vi "startTest.vi"(8 "error in (no error)":errorcluster, 10 "test":refnum<class>, 11 "TestResult in":refnum<class "TestResult.lvclass">) -> (0 "error out":errorcluster, 3 "TestResult in":refnum<class "TestResult.lvclass">)   [LabVIEW 2013, in "TestResult.lvclass"]
uses:
  TestResult.lvclass
  testStarted--Cluster.ctl
  TestResult.lvclass/TestResult.ctl
panel:
  # "JKI VI Tester for LabVIEW\nhttp://jkisoft.com/vi-tester\nCopyright (C) 2007-2009, JKI <info@jkisoft.com>\nALL RIGHTS RESERVED"
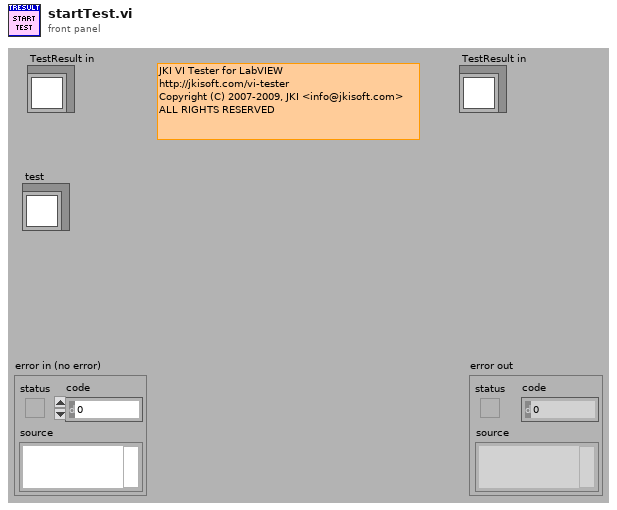
[diagram p1: front panel]
types:
  T1 = typedef "TestResult.lvclass/testStarted--Cluster.ctl" = cluster{"test":refnum<class>, "startTimestamp":timestamp}
  T2 = typedef "TestResult.lvclass/testsRun.ctl" = u32
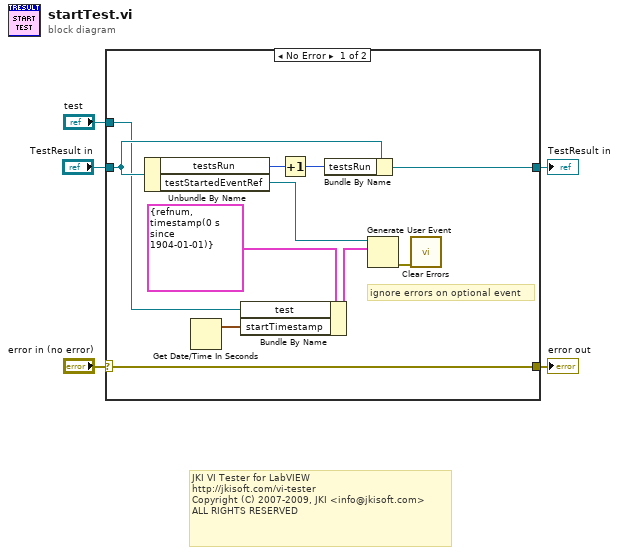
[diagram p0: block diagram]
diagram:
  # "JKI VI Tester for LabVIEW\nhttp://jkisoft.com/vi-tester\nCopyright (C) 2007-2009, JKI <info@jkisoft.com>\nALL RIGHTS RESERVED"
  n1 = case shown="No Error" "error in (no error)" {
    selector: "error in (no error)" -> [w15 w18]
    tunnel: [w15 w18] -> w4
    tunnel: [w13 w17] -> w2
    tunnel: "TestResult in" -> [w14 w17]
    tunnel: "test" -> [w8 _]
    frame No Error {
      # "ignore errors on optional event"
      n2 = Unbundle By Name(w14) -> ("testsRun"=w16:T2, "testStartedEventRef"=w11:refnum<user-event>)
      n3 = Get Date/Time In Seconds() -> (seconds since 1Jan1904=w7:timestamp)
      n4 = Bundle By Name(cluster=T1 {"test"=refnum, "startTimestamp"=timestamp(0 s since 1904-01-01)} ("event data"), "test"=w8, "startTimestamp"=w7) -> (w9:T1)
      n5 = Increment(x=w16) -> (x+1=w12:T2)
      n6 = Bundle By Name(cluster=w14, "testsRun"=w12) -> (w13:refnum<class "TestResult.lvclass">)
      n7 = Generate User Event(user event=w11, event data cluster=w9) -> (error out=w6:errorcluster)  [unwired: 2 in, 1 out]
      n8 = call <vilib>:"Clear Errors.vi"("error in (no error)"=w6) -> ()  [unwired: 6 in, 1 out]
    }
    frame Error {
    }
  }
  "error out" <- w4
  "TestResult in" <- w2
